vi "Get Scope Error IDs.vi"(7 "scope":T1, 8 "error in (no error)":errorcluster, 11 "error list <top>":variant) -> (0 "error out":errorcluster, 2 "error IDs":T2[](array[typedef]), 3 "error list <top> dup":variant)   [LabVIEW 2017]
uses:
  Error Owner and ID.ctl
  Scope.ctl
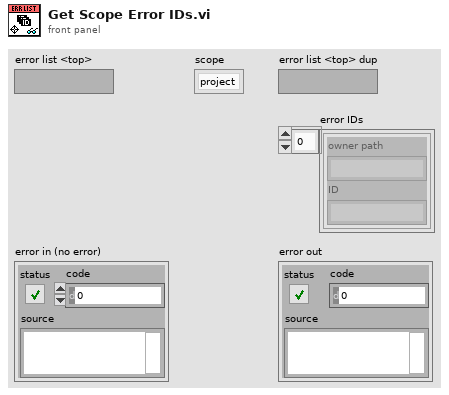
[diagram p1: front panel]
types:
  T1 = typedef "Scope.ctl" = enum16{"project", "global"}
  T2 = typedef "Error Owner and ID.ctl" = cluster{"owner path":string, "ID":string}
  T3 = typedef "Error File Management.lvlib/NI Error.ctl" = errorcluster
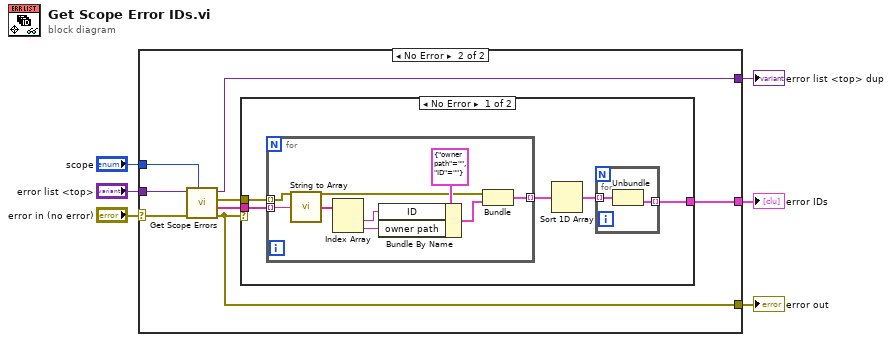
[diagram p0: block diagram]
diagram:
  n1 = case shown="No Error" "error in (no error)" {
    selector: "error in (no error)" -> [w8 w13]
    tunnel: [_ w14] -> w6
    tunnel: [w8 w15] -> w4
    tunnel: "error list <top>" -> [w7 w12]
    tunnel: "scope" -> [_ w11]
    tunnel: [w7 w10] -> w1
    frame Error {
    }
    frame No Error {
      n2 = call "Get Scope Errors.vi"("scope"=w11, "error in (no error)"=w13, "error list <top> in"=w12) -> ("error out"=w15:errorcluster, "attributes"=w16:string[], "errors"=w9:T3[], "error list <top> out"=w10:variant)  [unwired: 4 in, 1 out]
      n3 = case shown="No Error" w15 {
        tunnel: w16 -> [w21 _]
        tunnel: [w17 _] -> w14
        tunnel: w9 -> [w20 _]
        frame No Error {
          n4 = for {
            tunnel: w21 -> [w31] mode=indexing
            tunnel: w20 -> [w25] mode=indexing
            tunnel: [w24] -> w19 mode=indexing
            n5 = call "String to Array.vi"("string"=w31) -> ("array"=w30:string[])  [unwired: 1 in]
            n6 = Index Array(array=w30) -> (element #1=w28:string, element #2=w27:string)  [unwired: 2 in]
            n7 = Bundle By Name(cluster=T2 {"owner path"="", "ID"=""} ("owner error"), "ID"=w28, "owner path"=w27) -> (w26:T2)
            n8 = Bundle("error"=w25, "owner error"=w26) -> (w24:cluster{"error":T3, "owner error":T2})  [unwired: 1 in]
          }
          n9 = Sort 1D Array(array=w19) -> (sorted array=w18:cluster{"error":T3, "owner error":T2}[])
          n10 = for {
            tunnel: w18 -> [w23] mode=indexing
            tunnel: [w22] -> w17 mode=indexing
            n11 = Unbundle(w23) -> ("owner error"=w22:T2)  [unwired: 1 out]
          }
        }
        frame Error {
        }
      }
    }
  }
  "error IDs" <- w6
  "error out" <- w4
  "error list <top> dup" <- w1
